vi "Initiate assembly_12042024.vi"(0 "Database Entry in":refnum<class "Database Entry.lvclass">, 11 "error in (no error)":errorcluster) -> (2 "Feet check":bool, 3 "PUT Settings":T1(array[cluster]), 4 "Database Entry out":refnum<class "Database Entry.lvclass">, 6 "Module?":bool, 8 "Abort out":bool, 10 "Assembly Settings":T1(array[cluster]), 12 "Assembly Type":string[](array[string]), 13 "Stack names":string[](array[string]), 14 "Component Settings":T1(array[cluster]), 15 "error out":errorcluster)   [LabVIEW 2021, in "Database Entry.lvclass"]
uses:
  Database Entry.lvclass
  Database Entry.lvclass/Database Entry.ctl
  <vilib>/Utility/file.llb/Read Delimited Spreadsheet (string).vi
  Components/Stack/Stack.lvclass
  <vilib>/JDP Science/JDP Science Common Utilities/JDP Utility.lvlib
panel:
  out "Now assembling...":string
  in  "Abort":bool
  in  "Relative humidity":string
  in  "Temperature (C)":string
  in  "ROC version":u16(ring)=1 items=["HGCROCV3b-2", "HGCROCV3b-4", "HGCROCV3c", "Preseries"]
  in  "Adhesive":u16(ring) items=["Hybrid", "Transfer tape only", "Epoxy only"]
  in  "Module Type":u16(ring) items=["CMU,LD,Full,200,CuW", "CMU,LD,Full,300,CuW", "CMU,LD,Full,200,Ti", "CMU,LD,Full,300,Ti", "CMU,LD,Full,200,CF", "CMU,LD,Full,300,CF"]
  in  "Operator":u16(ring) items=["jestein", "simurthy", "cmumac"]
  out "Selected postitions":dbl[](array[numeric])
  out "Status":dbl[][](array[numeric])
  in  "Assembly Region":cluster{"1":bool, "2":bool, "3":bool, "4":bool}
  in  "Submit":bool
  # "Tray Slot 1"
  # "Tray Slot 2"
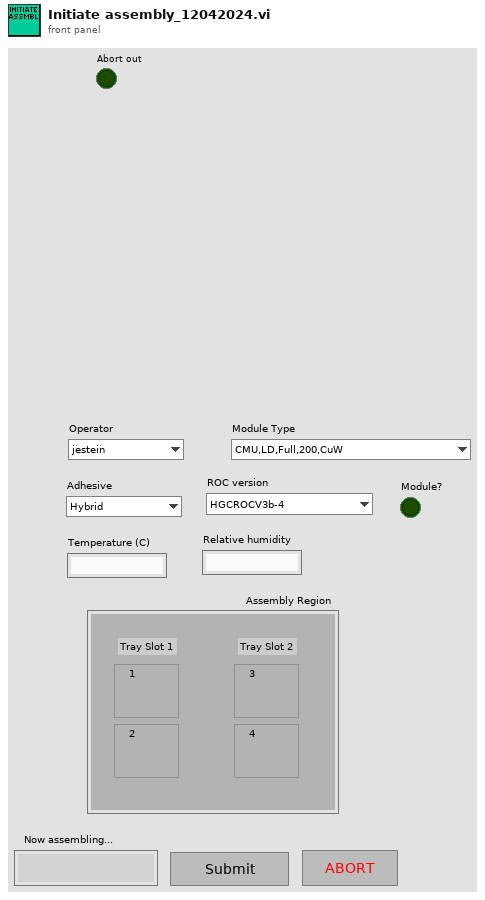
[diagram p1: front panel]
types:
  T1 = cluster{"Fixture ID":dbl, "Position":dbl, "Thickness":dbl}[]
  T2 = typedef "File Paths.ctl" = cluster{"Glue Pattern Folder":path, "Carrier Tray Folder":path, "Pick Up Tool Fixture Folder":path, "Components Folder":path, "Bellows Tool Offset.txt":path, "Pick Up Tool Offset.txt":path, "Dispense Tip Offset.txt":path, "Log Files":path, "Gantry Assembly Map.txt":path, "Syringe and offset map.txt":path, "Controllers Folder":path, "Local dbase config":path}
  T3 = cluster{"Temperature (C)":string, "Relative humidity":string}
  T4 = cluster{"Fixture ID":dbl, "Position":dbl, "Thickness":dbl}
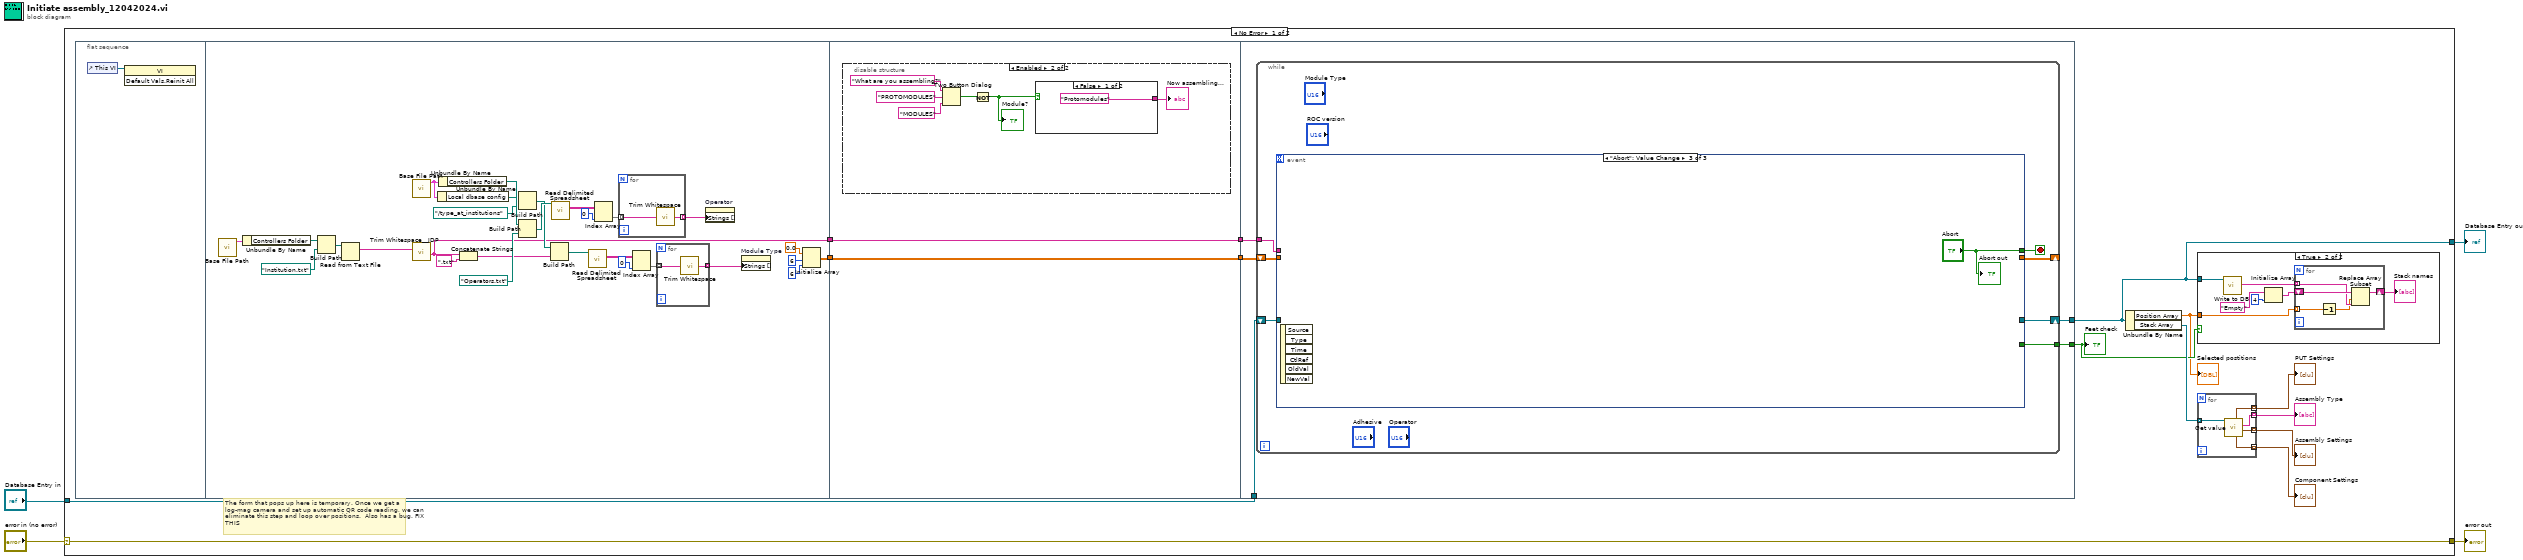
[diagram p0: block diagram]
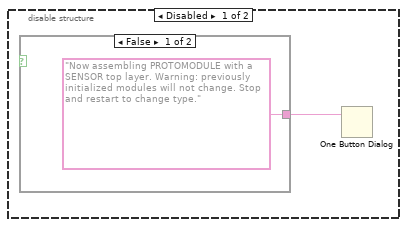
[diagram p3: hidden frame]
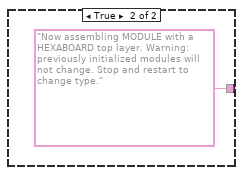
[diagram p4: hidden frame]
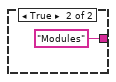
[diagram p5: hidden frame]
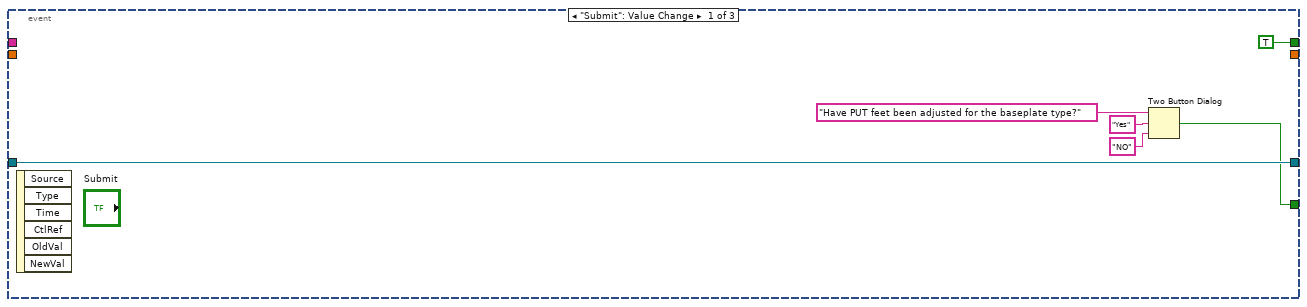
[diagram p6: hidden frame]
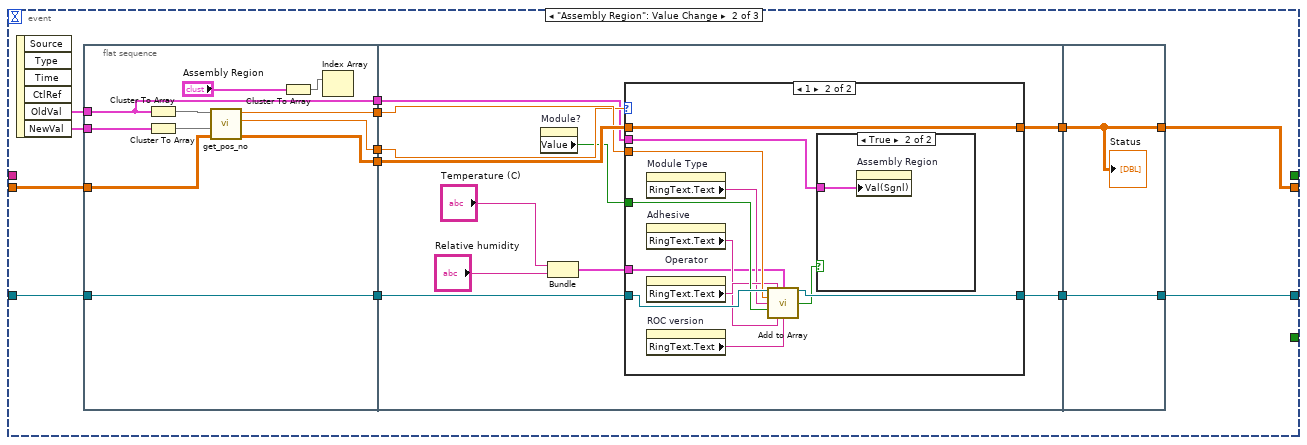
[diagram p7: hidden frame]
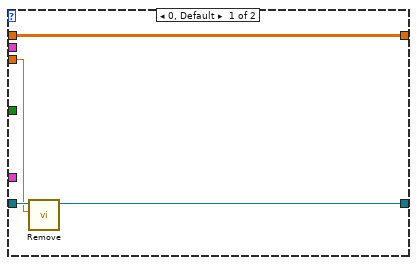
[diagram p8: hidden frame]
diagram:
  n1 = case shown="No Error" "error in (no error)" {
    selector: "error in (no error)" -> [w18 w156]
    tunnel: [w18 w156] -> w3
    tunnel: [w16 w155] -> w1
    tunnel: "Database Entry in" -> [w17 w155]
    frame No Error {
      # "The form that pops up here is temporary. Once we get a log-mag camera and set up automatic QR code reading, we can eliminate this step and loop over positions.  Also has a bug. FIX THIS"
      n2 = flat-sequence {
        tunnel: [w55] -> w8
        tunnel: [w44] -> w6
        tunnel: w8 -> [w70]
        tunnel: [w70] -> w7
        tunnel: w6 -> [w69]
        tunnel: [w69] -> w5
        tunnel: w7 -> [w85]
        tunnel: w5 -> [w84]
        tunnel: w17 -> [w86]
        tunnel: [w83] -> w16
        tunnel: [w82] -> w10
        frame #0 {
          n3 = control-ref of="This VI"() -> (w36:refnum<vi>)
          n4 = invoke class="VI" method="Default Vals.Reinit All"(reference=w36) -> ()  [unwired: 2 in, 3 out]
        }
        frame #1 {
          n5 = call "Base File Path.vi"() -> ("Paths Out"=w64:T2)  [unwired: 11 in]
          n6 = Unbundle By Name(w64) -> ("Controllers Folder"=w46:path)
          n7 = Build Path(base path=w46, name or relative path=path "Institution.txt") -> (appended path=w62:path)
          n8 = Read from Text File(file (use dialog)=w62) -> (text=w61:string)  [unwired: 3 in, 3 out]
          n9 = call "Base File Path.vi"() -> ("Paths Out"=w51:T2)  [unwired: 11 in]
          n10 = call <vilib>:"Trim Whitespace__JDP.vi"("String in"=w61) -> ("String out"=w44:string)  [unwired: 6 in]
          n11 = Unbundle By Name(w51) -> ("Local dbase config"=w50:path)
          n12 = Unbundle By Name(w51) -> ("Controllers Folder"=w60:path)
          n13 = Concatenate Strings(w44, ".txt" ("string")) -> (w42:string)
          n14 = Build Path(base path=w50, name or relative path=path "../type_at_institutions") -> (appended path=w47:path)
          n15 = Build Path(base path=w60, name or relative path=path "Operators.txt") -> (appended path=w58:path)
          n16 = Build Path(base path=w47, name or relative path=w42) -> (appended path=w45:path)
          n17 = call-poly <vilib>:"Read Delimited Spreadsheet.vi"("file path (dialog if empty)"=w58) -> ("all rows"=w57:string[][])  [unwired: 9 in, 5 out]
          n18 = call-poly <vilib>:"Read Delimited Spreadsheet.vi"("file path (dialog if empty)"=w45) -> ("all rows"=w41:string[][])  [unwired: 9 in, 5 out]
          n19 = Index Array(array=w57, index (col)=0 ("disabled index (col)")) -> (element=w40:string[])  [unwired: 1 in]
          n20 = for {
            tunnel: w40 -> [w68] mode=indexing
            tunnel: [w67] -> w39 mode=indexing
            n21 = call <vilib>:"Trim Whitespace.vi"("string"=w68) -> ("trimmed string"=w67:string)  [unwired: 1 in]
          }
          n22 = Index Array(array=w41, index (col)=0 ("disabled index (col)")) -> (element=w38:string[])  [unwired: 1 in]
          n23 = for {
            tunnel: w38 -> [w66] mode=indexing
            tunnel: [w65] -> w37 mode=indexing
            n24 = call <vilib>:"Trim Whitespace.vi"("string"=w66) -> ("trimmed string"=w65:string)  [unwired: 1 in]
          }
          n25 = property on="Operator" class="Ring (strict)"("Strings []"=w39) -> ()  [unwired: 2 in, 2 out]
          n26 = property on="Module Type" class="Ring (strict)"("Strings []"=w37) -> ()  [unwired: 2 in, 2 out]
          n27 = Initialize Array(0.0 ("element"), 6 ("dimension size"), 6 ("dimension size")) -> (w55:dbl[][])
        }
        frame #2 {
          n28 = disable-structure shown="Enabled" {
            frame Disabled {
              n29 = case shown="False" {
                selector: _ -> [_ _]
                tunnel: ["Now assembling PROTOMODULE with a SENSOR top layer. Warning: previously initialized modules will not change. Stop and restart to change type." "Now assembling MODULE with a HEXABOARD top layer. Warning: previously initialized modules will not change. Stop and restart to change type."] -> w71
                frame False {
                }
                frame True {
                }
              }
              n30 = One Button Dialog(message=w71) -> ()  [unwired: 1 in, 1 out]
            }
            frame Enabled {
              n31 = Two Button Dialog(message="What are you assembling?", 1:"MODULES" ("F button name (\"Cancel\")"), 2:"PROTOMODULES" ("T button name (\"OK\")")) -> (T button?=w76:bool)
              n32 = Not(x=w76) -> (.not. x?=w75:bool)
              "Module?" <- w75
              n33 = case shown="False" w75 {
                tunnel: ["Protomodules" ("Now assembling...") "Modules" ("Now assembling...")] -> w74
                frame False {
                }
                frame True {
                }
              }
              "Now assembling..." <- w74
            }
          }
        }
        frame #3 {
          n34 = while {
            shift-right: [w93] -> w83
            shift-left: w86 -> [w90]
            shift-right: [w91] -> _
            shift-left: w85 -> [w92]
            tunnel: w84 -> [w89]
            tunnel: [w87] -> w82
            stop <- w88 stop-if-true
            n35 = event shown="[2] \"Abort\": Value Change" {
              selector: _ -> [_ _ _]
              dyn-events: _ -> [_ _ _]
              timeout: _ -> [_ _ _]
              tunnel: [TRUE ("T button?") _ "Abort"] -> w88
              tunnel: w90 -> [w99 w106 _]
              tunnel: [w99 w103 _] -> w93
              tunnel: w92 -> [_ w111 _]
              tunnel: [_ w107 _] -> w91
              tunnel: w89 -> [_ _ _]
              tunnel: [w94 _ _] -> w87
              event "Submit": Value Change {
                n36 = event-data() -> ()  [unwired: 1 in, 6 out]
                n37 = Two Button Dialog(message="Have PUT feet been adjusted for the baseplate type?", 1:"NO" ("F button name (\"Cancel\")"), 2:"Yes" ("T button name (\"OK\")")) -> (T button?=w94:bool)
              }
              event "Assembly Region": Value Change {
                n38 = event-data() -> ("OldVal"=w100:cluster{"1":bool, "2":bool, "3":bool, "4":bool}, "NewVal"=w112:cluster{"1":bool, "2":bool, "3":bool, "4":bool})  [unwired: 1 in, 4 out]
                n39 = flat-sequence {
                  tunnel: w112 -> [w122]
                  tunnel: w100 -> [w113]
                  tunnel: w111 -> [w118]
                  tunnel: [w115] -> w109
                  tunnel: [w117] -> w108
                  tunnel: w106 -> [w116]
                  tunnel: [w116] -> w105
                  tunnel: [w114] -> w104
                  tunnel: [w113] -> w101
                  tunnel: [w133] -> w110
                  tunnel: w109 -> [w134]
                  tunnel: w108 -> [w131]
                  tunnel: w105 -> [w132]
                  tunnel: w104 -> [w130]
                  tunnel: [w129] -> w102
                  tunnel: w101 -> [w128]
                  tunnel: w110 -> [w153]
                  tunnel: [w153] -> w107
                  tunnel: [w152] -> w103
                  tunnel: w102 -> [w152]
                  frame #0 {
                    n40 = Cluster To Array(cluster=w113) -> (array=w119:bool[])
                    n41 = Cluster To Array(cluster=w122) -> (array=w120:bool[])
                    n42 = call "get_pos_no.vi"("Status Old"=w118, "Array New Status"=w120, "Array Old Status"=w119) -> ("Status New"=w115:dbl[][], "State"=w114:dbl, "Position ID"=w117:dbl)  [unwired: 2 in]
                    n43 = Cluster To Array(cluster="Assembly Region") -> (array=w123:bool[])
                    n44 = Index Array(array=w123) -> ()  [unwired: 1 in, 1 out]
                  }
                  frame #1 {
                    n45 = property on="Module?" class="Bool (strict)"() -> ("Value"=w127:bool)  [unwired: 2 in, 2 out]
                    n46 = Bundle("Temperature (C)"="Temperature (C)", "Relative humidity"="Relative humidity") -> (w124:T3)  [unwired: 1 in]
                    n47 = case shown="1" w130 {
                      tunnel: w134 -> [w135 w150]
                      tunnel: [w135 w150] -> w133
                      tunnel: w132 -> [w138 w149]
                      tunnel: [w137 w148] -> w129
                      tunnel: w131 -> [w136 w147]
                      tunnel: w127 -> [_ w146]
                      tunnel: w128 -> [_ w140]
                      tunnel: w124 -> [_ w139]
                      frame 0, Default {
                        n48 = call "Remove.vi"("Index"=w136, "Database Entry in"=w138) -> ("Database Entry out"=w137:refnum<class "Database Entry.lvclass">)  [unwired: 8 in, 1 out]
                      }
                      frame 1 {
                        n49 = property on="Module Type" class="Ring (strict)"() -> ("RingText.Text"=w144:string)  [unwired: 2 in, 2 out]
                        n50 = property on="Adhesive" class="Ring (strict)"() -> ("RingText.Text"=w143:string)  [unwired: 2 in, 2 out]
                        n51 = property on="Operator" class="Ring (strict)"() -> ("RingText.Text"=w145:string)  [unwired: 2 in, 2 out]
                        n52 = property on="ROC version" class="Ring (strict)"() -> ("RingText.Text"=w142:string)  [unwired: 2 in, 2 out]
                        n53 = call "Add to Array.vi"("Database Entry in"=w149, "Operator"=w145, "Temp and RelHumidity"=w139, "Position Index"=w147, "Module type"=w144, "Module?"=w146, "Adhesive"=w143, "ROC version"=w142) -> ("Database Entry out"=w148:refnum<class "Database Entry.lvclass">, "Position cancelled?"=w141:bool)  [unwired: 5 in, 1 out]
                        n54 = case shown="True" w141 {
                          tunnel: w140 -> [_ w151]
                          frame False {
                          }
                          frame True {
                            n55 = property on="Assembly Region" class="Clust (strict)"("Val(Sgnl)"=w151) -> ()  [unwired: 2 in, 2 out]
                          }
                        }
                      }
                    }
                  }
                  frame #2 {
                    "Status" <- w153
                  }
                }
              }
              event "Abort": Value Change {
                n56 = event-data() -> ()  [unwired: 1 in, 6 out]
                "Abort out" <- "Abort"
              }
            }
          }
        }
      }
      n57 = Unbundle By Name(w16) -> ("Position Array"=w9:dbl[], "Stack Array"=w15:refnum<class "Stack.lvclass">[])
      "Selected postitions" <- w9
      n58 = case shown="True" w10 {
        tunnel: w16 -> [_ w25]
        tunnel: w9 -> [_ w24]
        frame False {
        }
        frame True {
          n59 = call "Write to DB.vi"("Database Entry in"=w25) -> ("Stack names"=w19:string[])  [unwired: 8 in, 2 out]
          n60 = Initialize Array("Empty", 4 ("dimension size")) -> (w20:string[])
          n61 = for {
            tunnel: w24 -> [w28] mode=indexing
            tunnel: w19 -> [w29] mode=indexing
            shift-right: [w26] -> w23
            shift-left: w20 -> [w30]
            n62 = Decrement(x=w28) -> (x-1=w27:dbl)
            n63 = Replace Array Subset(array=w30, new element=w29, index=w27) -> (w26:string[])
          }
          "Stack names" <- w23
        }
      }
      n64 = for {
        tunnel: w15 -> [w35] mode=indexing
        tunnel: [w34] -> w14 mode=indexing
        tunnel: [w33] -> w13 mode=indexing
        tunnel: [w32] -> w12 mode=indexing
        tunnel: [w31] -> w11 mode=indexing
        n65 = call "Get value.vi"("Stack in"=w35) -> ("Assembly Settings"=w32:T4, "Resolution Geometry"=w31:string, "Component Settings"=w33:T4, "PUT Settings"=w34:T4)  [unwired: 5 in, 2 out]
      }
      "Assembly Settings" <- w12
      "Component Settings" <- w13
      "PUT Settings" <- w14
      "Assembly Type" <- w11
      "Feet check" <- w10
    }
    frame Error {
    }
  }
  "error out" <- w3
  "Database Entry out" <- w1
